vi "GDSLvIcon_BuildPictureRows.vi"(1 "RowTextPictures":cluster{"RowPict":bool[][]}[](array[cluster])=[{"RowPict"=[[FALSE, TRUE, TRUE, TRUE, FALSE, TRUE, TRUE, FALSE, FALSE, TRUE, FALSE], [TRUE, FALSE, FALSE, TRUE, FALSE, TRUE, FALSE, FALSE, FALSE, TRUE, FALSE], [TRUE, FALSE, TRUE, TRUE, FALSE, TRUE, TRUE, FALSE, FALSE, TRUE, FALSE], [TRUE, FALSE, FALSE, FALSE, FALSE, TRUE, FALSE, FALSE, FALSE, TRUE, FALSE], [FALSE, TRUE, TRUE, TRUE, FALSE, TRUE, TRUE, FALSE, TRUE, TRUE, TRUE]]}, {"RowPict"=[[TRUE, TRUE, FALSE, FALSE, TRUE, FALSE, TRUE, FALSE, FALSE, TRUE, FALSE, FALSE, TRUE, FALSE, TRUE], [TRUE, FALSE, TRUE, FALSE, TRUE, FALSE, TRUE, FALSE, FALSE, TRUE, FALSE, FALSE, TRUE, FALSE, TRUE], [TRUE, FALSE, TRUE, FALSE, TRUE, TRUE, TRUE, FALSE, FALSE, TRUE, FALSE, FALSE, TRUE, TRUE, TRUE], [TRUE, FALSE, TRUE, FALSE, TRUE, FALSE, TRUE, FALSE, FALSE, TRUE, FALSE, FALSE, TRUE, FALSE, TRUE], [TRUE, TRUE, FALSE, FALSE, FALSE, TRUE, FALSE, FALSE, TRUE, TRUE, TRUE, FALSE, FALSE, TRUE, FALSE]]}], 2 "Pixel width":i32=30, 3 "Alignment":T1, 4 "Offset":cluster{"X":i32, "Y":i32}, 5 "error in (no error)":errorcluster, 6 "Pixel height":i32=22) -> (15 "CharPicture":bool[][](array[boolean])=[[FALSE, FALSE, FALSE, FALSE, FALSE, FALSE, FALSE, FALSE, FALSE, FALSE, FALSE, FALSE, FALSE, FALSE, FALSE, FALSE, FALSE, FALSE, FALSE, FALSE, FALSE, FALSE, FALSE, FALSE, FALSE, FALSE, FALSE, FALSE, FALSE, FALSE], [FALSE, FALSE, FALSE, FALSE, FALSE, FALSE, FALSE, FALSE, FALSE, FALSE, FALSE, FALSE, FALSE, FALSE, FALSE, FALSE, FALSE, FALSE, FALSE, FALSE, FALSE, FALSE, FALSE, FALSE, FALSE, FALSE, FALSE, FALSE, FALSE, FALSE], [FALSE, FALSE, FALSE, FALSE, FALSE, FALSE, FALSE, FALSE, FALSE, FALSE, FALSE, FALSE, FALSE, FALSE, FALSE, FALSE, FALSE, FALSE, FALSE, FALSE, FALSE, FALSE, FALSE, FALSE, FALSE, FALSE, FALSE, FALSE, FALSE, FALSE], [FALSE, FALSE, FALSE, FALSE, FALSE, FALSE, FALSE, FALSE, FALSE, FALSE, FALSE, FALSE, FALSE, FALSE, FALSE, FALSE, FALSE, FALSE, FALSE, FALSE, FALSE, FALSE, FALSE, FALSE, FALSE, FALSE, FALSE, FALSE, FALSE, FALSE], [FALSE, FALSE, FALSE, FALSE, FALSE, FALSE, FALSE, FALSE, FALSE, FALSE, FALSE, FALSE, FALSE, FALSE, FALSE, FALSE, FALSE, FALSE, FALSE, FALSE, TRUE, TRUE, TRUE, FALSE, TRUE, TRUE, FALSE, TRUE, TRUE, TRUE], [FALSE, FALSE, FALSE, FALSE, FALSE, FALSE, FALSE, FALSE, FALSE, FALSE, FALSE, FALSE, FALSE, FALSE, FALSE, FALSE, FALSE, FALSE, FALSE, TRUE, FALSE, FALSE, FALSE, FALSE, TRUE, FALSE, FALSE, FALSE, TRUE, FALSE], [FALSE, FALSE, FALSE, FALSE, FALSE, FALSE, FALSE, FALSE, FALSE, FALSE, FALSE, FALSE, FALSE, FALSE, FALSE, FALSE, FALSE, FALSE, FALSE, TRUE, FALSE, TRUE, TRUE, FALSE, TRUE, TRUE, FALSE, FALSE, TRUE, FALSE], [FALSE, FALSE, FALSE, FALSE, FALSE, FALSE, FALSE, FALSE, FALSE, FALSE, FALSE, FALSE, FALSE, FALSE, FALSE, FALSE, FALSE, FALSE, FALSE, TRUE, FALSE, FALSE, TRUE, FALSE, TRUE, FALSE, FALSE, FALSE, TRUE, FALSE], [FALSE, FALSE, FALSE, FALSE, FALSE, FALSE, FALSE, FALSE, FALSE, FALSE, FALSE, FALSE, FALSE, FALSE, FALSE, FALSE, FALSE, FALSE, FALSE, FALSE, TRUE, TRUE, TRUE, FALSE, TRUE, TRUE, FALSE, FALSE, TRUE, FALSE], [FALSE, FALSE, FALSE, FALSE, FALSE, FALSE, FALSE, FALSE, FALSE, FALSE, FALSE, FALSE, FALSE, FALSE, FALSE, FALSE, FALSE, FALSE, FALSE, FALSE, FALSE, FALSE, FALSE, FALSE, FALSE, FALSE, FALSE, FALSE, FALSE, FALSE], [FALSE, FALSE, FALSE, FALSE, FALSE, FALSE, FALSE, FALSE, FALSE, FALSE, FALSE, FALSE, FALSE, FALSE, FALSE, FALSE, FALSE, FALSE, FALSE, FALSE, FALSE, FALSE, FALSE, FALSE, FALSE, FALSE, FALSE, FALSE, FALSE, FALSE], [FALSE, FALSE, FALSE, FALSE, FALSE, FALSE, FALSE, FALSE, FALSE, FALSE, FALSE, FALSE, FALSE, FALSE, FALSE, FALSE, FALSE, FALSE, FALSE, FALSE, FALSE, FALSE, FALSE, FALSE, FALSE, FALSE, FALSE, FALSE, FALSE, FALSE], [FALSE, FALSE, FALSE, FALSE, FALSE, FALSE, FALSE, FALSE, FALSE, FALSE, FALSE, FALSE, FALSE, FALSE, FALSE, FALSE, FALSE, FALSE, FALSE, FALSE, FALSE, FALSE, FALSE, FALSE, FALSE, FALSE, FALSE, FALSE, FALSE, FALSE], [FALSE, FALSE, FALSE, FALSE, FALSE, FALSE, FALSE, FALSE, FALSE, FALSE, FALSE, FALSE, FALSE, FALSE, FALSE, TRUE, TRUE, FALSE, FALSE, FALSE, TRUE, FALSE, FALSE, TRUE, TRUE, TRUE, FALSE, FALSE, TRUE, FALSE], [FALSE, FALSE, FALSE, FALSE, FALSE, FALSE, FALSE, FALSE, FALSE, FALSE, FALSE, FALSE, FALSE, FALSE, FALSE, TRUE, FALSE, TRUE, FALSE, TRUE, FALSE, TRUE, FALSE, FALSE, TRUE, FALSE, FALSE, TRUE, FALSE, TRUE], [FALSE, FALSE, FALSE, FALSE, FALSE, FALSE, FALSE, FALSE, FALSE, FALSE, FALSE, FALSE, FALSE, FALSE, FALSE, TRUE, FALSE, TRUE, FALSE, TRUE, TRUE, TRUE, FALSE, FALSE, TRUE, FALSE, FALSE, TRUE, TRUE, TRUE], [FALSE, FALSE, FALSE, FALSE, FALSE, FALSE, FALSE, FALSE, FALSE, FALSE, FALSE, FALSE, FALSE, FALSE, FALSE, TRUE, FALSE, TRUE, FALSE, TRUE, FALSE, TRUE, FALSE, FALSE, TRUE, FALSE, FALSE, TRUE, FALSE, TRUE], [FALSE, FALSE, FALSE, FALSE, FALSE, FALSE, FALSE, FALSE, FALSE, FALSE, FALSE, FALSE, FALSE, FALSE, FALSE, TRUE, TRUE, FALSE, FALSE, TRUE, FALSE, TRUE, FALSE, FALSE, TRUE, FALSE, FALSE, TRUE, FALSE, TRUE], [FALSE, FALSE, FALSE, FALSE, FALSE, FALSE, FALSE, FALSE, FALSE, FALSE, FALSE, FALSE, FALSE, FALSE, FALSE, FALSE, FALSE, FALSE, FALSE, FALSE, FALSE, FALSE, FALSE, FALSE, FALSE, FALSE, FALSE, FALSE, FALSE, FALSE], [FALSE, FALSE, FALSE, FALSE, FALSE, FALSE, FALSE, FALSE, FALSE, FALSE, FALSE, FALSE, FALSE, FALSE, FALSE, FALSE, FALSE, FALSE, FALSE, FALSE, FALSE, FALSE, FALSE, FALSE, FALSE, FALSE, FALSE, FALSE, FALSE, FALSE], [FALSE, FALSE, FALSE, FALSE, FALSE, FALSE, FALSE, FALSE, FALSE, FALSE, FALSE, FALSE, FALSE, FALSE, FALSE, FALSE, FALSE, FALSE, FALSE, FALSE, FALSE, FALSE, FALSE, FALSE, FALSE, FALSE, FALSE, FALSE, FALSE, FALSE], [FALSE, FALSE, FALSE, FALSE, FALSE, FALSE, FALSE, FALSE, FALSE, FALSE, FALSE, FALSE, FALSE, FALSE, FALSE, FALSE, FALSE, FALSE, FALSE, FALSE, FALSE, FALSE, FALSE, FALSE, FALSE, FALSE, FALSE, FALSE, FALSE, FALSE]], 17 "X-Limited":bool, 18 "Y-Limited":bool, 19 "error out":errorcluster)   [LabVIEW 2020]
doc: "Puts the separate rows together to one picture. Each row is center and filled with spaces in the beginning and end."
uses:
  <resource>/Framework/Providers/Open_GDS/ClassProviders/Common/LvIcon_class/GDSLvIcon_TextAlignment.ctl
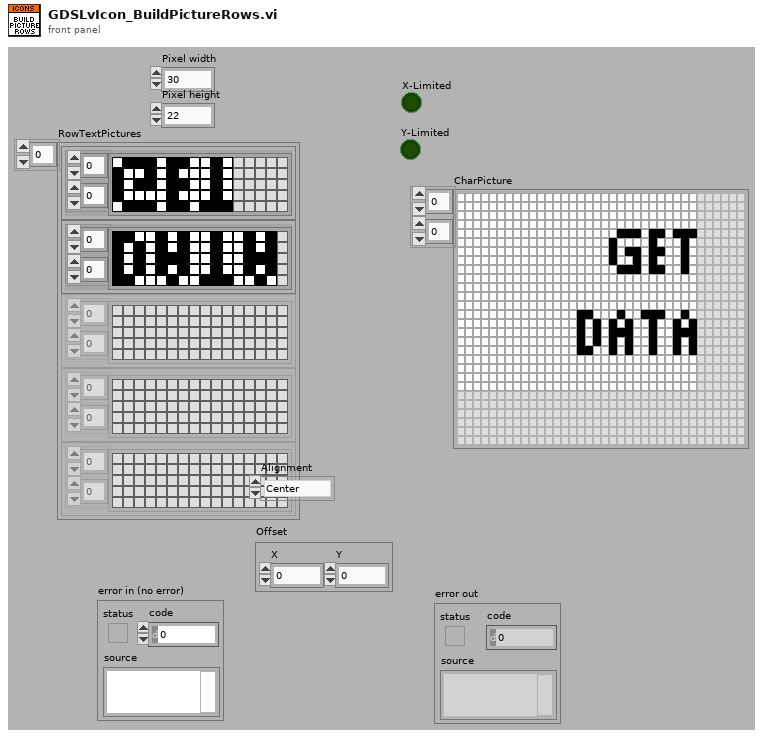
[diagram p1: front panel]
types:
  T1 = typedef "GDSLvIcon_TextAlignment.ctl" = enum16{"Center", "Left", "Right"}
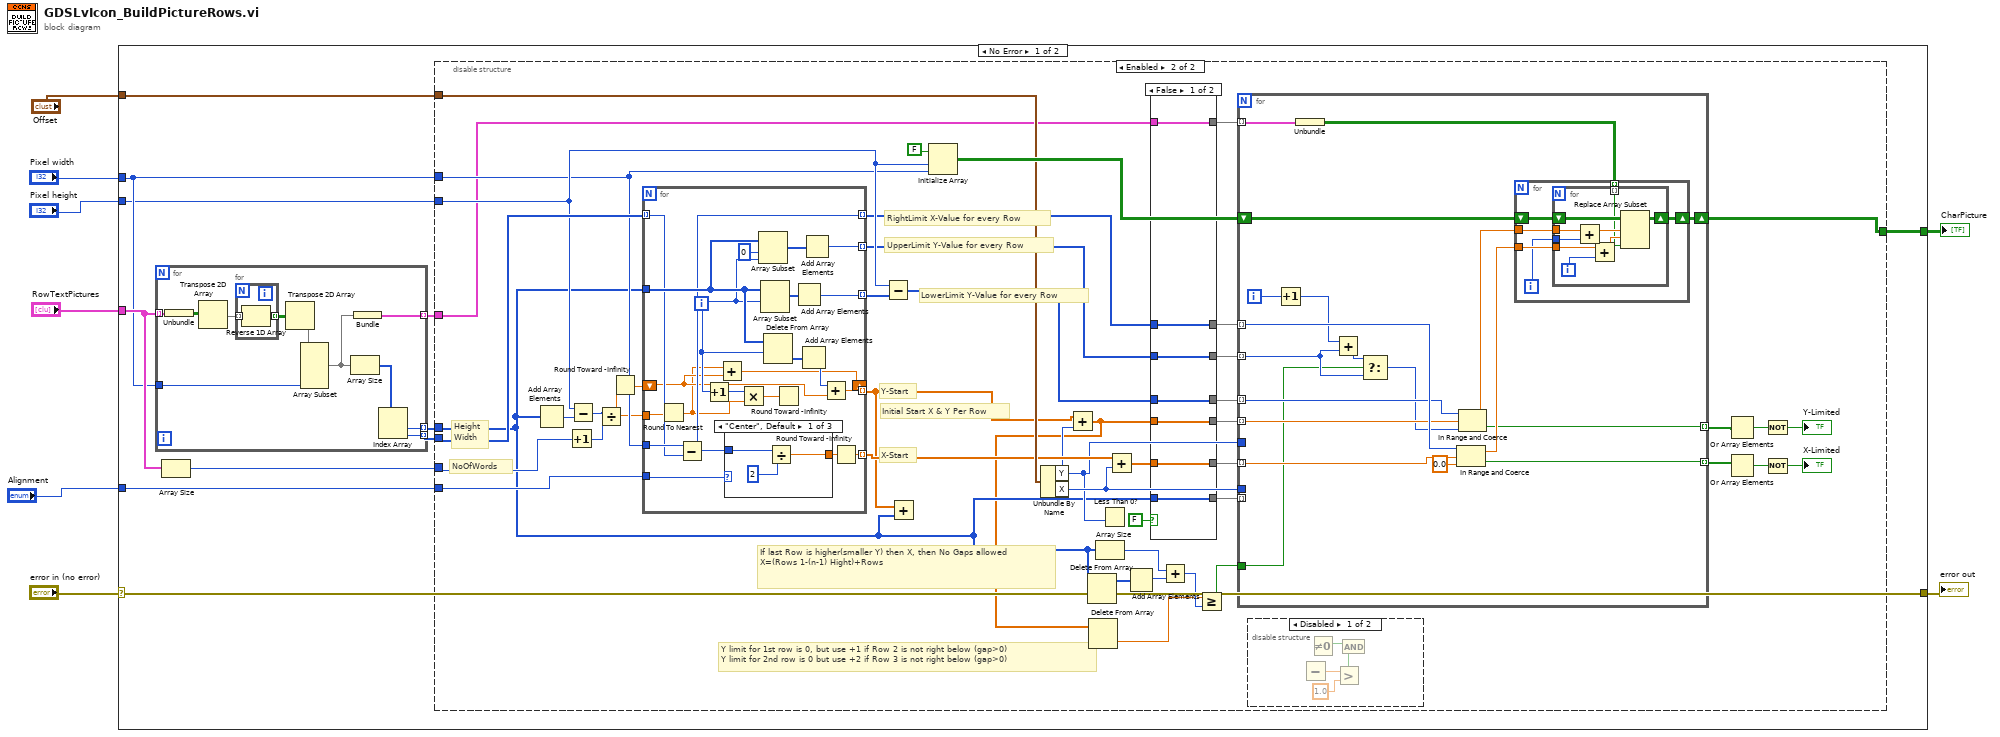
[diagram p0: block diagram]
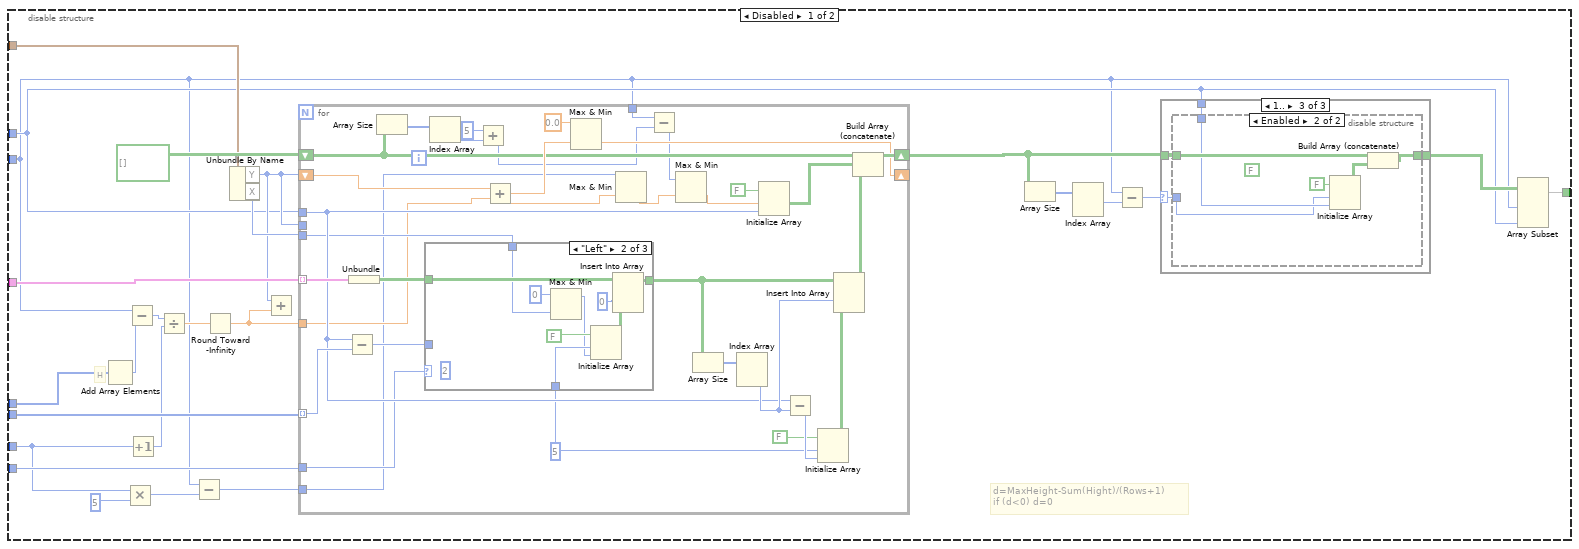
[diagram p2: hidden frame]
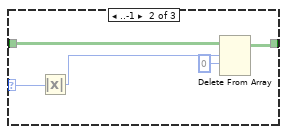
[diagram p4: hidden frame]
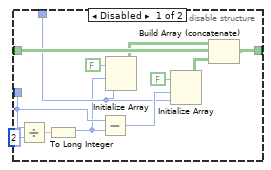
[diagram p5: hidden frame]
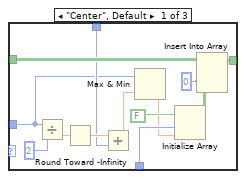
[diagram p6: hidden frame]
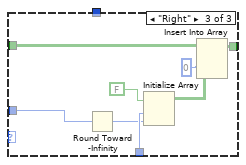
[diagram p7: hidden frame]
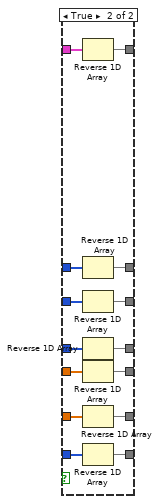
[diagram p9: hidden frame]
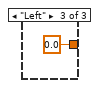
[diagram p11: hidden frame]
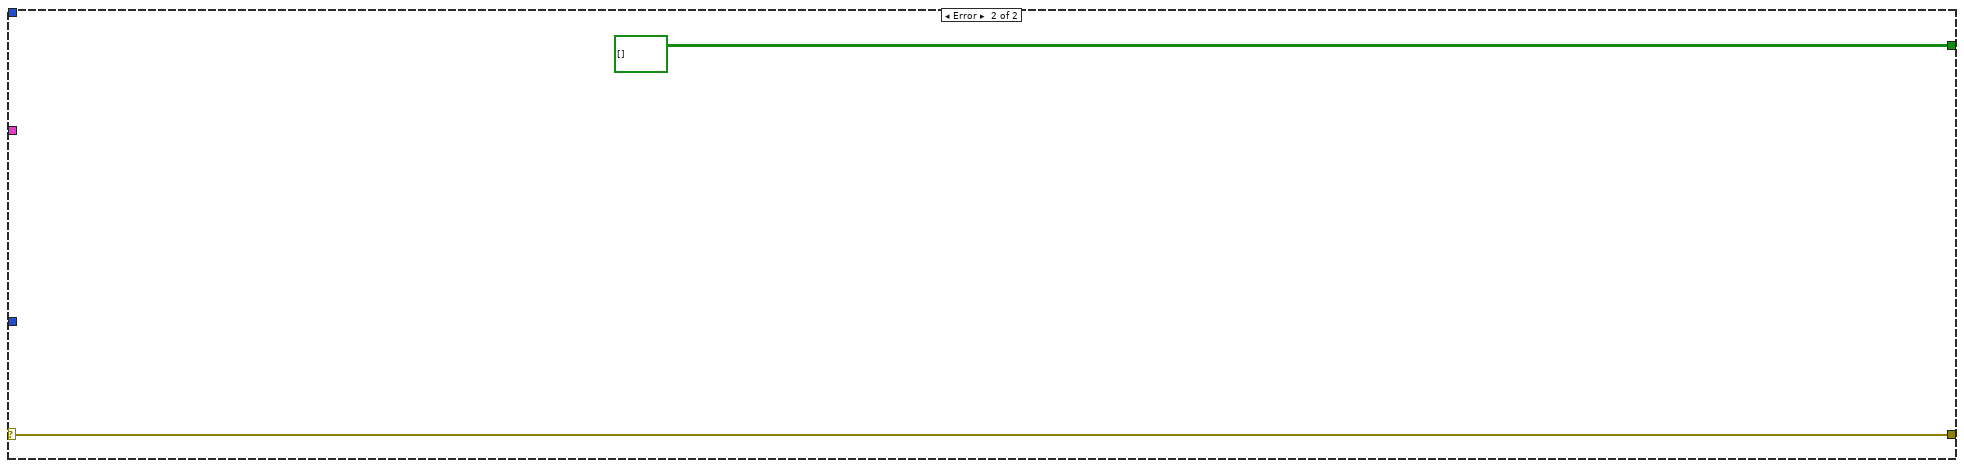
[diagram p12: hidden frame]
diagram:
  n1 = case shown="No Error" "error in (no error)" {
    selector: "error in (no error)" -> [w19 w282]
    tunnel: [w19 w282] -> w7
    tunnel: "Pixel width" -> [w11 _]
    tunnel: "RowTextPictures" -> [w15 _]
    tunnel: [w14 bool[][] [] ("CharPicture")] -> w5
    tunnel: "Pixel height" -> [w9 _]
    tunnel: "Alignment" -> [w13 _]
    tunnel: "Offset" -> [w12 _]
    frame No Error {
      n2 = for {
        tunnel: w15 -> [w275] mode=indexing
        tunnel: [w274] -> w17 mode=indexing
        tunnel: w11 -> [w273]
        tunnel: [w269] -> w18 mode=indexing
        tunnel: [w268] -> w16 mode=indexing
        n3 = Unbundle(w275) -> ("RowPict"=w276:bool[][])
        n4 = Transpose 2D Array(2D array=w276) -> (transposed array=w278:bool[][])
        n5 = for {
          tunnel: w278 -> [w280] mode=indexing
          tunnel: [w279] -> w277 mode=indexing
          n6 = Reverse 1D Array(array=w280) -> (reversed array=w279:bool[])
        }
        n7 = Transpose 2D Array(2D array=w277) -> (transposed array=w272:bool[][])
        n8 = Array Subset(array=w272, length (col)=w273) -> (w271:bool[][])  [unwired: 3 in]
        n9 = Array Size(array=w271) -> (size(s)=w270:i32[])
        n10 = Bundle(w271) -> (w274:cluster{bool[][]})  [unwired: 1 in]
        n11 = Index Array(array=w270) -> (element #1=w269:i32, element #2=w268:i32)  [unwired: 2 in]
      }
      n12 = Array Size(array=w15) -> (size(s)=w10:i32)
      n13 = disable-structure shown="Enabled" {
        disable-tunnel: w18 -> [w44 w140]
        disable-tunnel: w17 -> [w43 w156]
        disable-tunnel: w16 -> [w41 w178]
        disable-tunnel: [w37 w170] -> w14
        disable-tunnel: w13 -> [w36 w177]
        disable-tunnel: w12 -> [w34 w171]
        disable-tunnel: w11 -> [w25 w173]
        disable-tunnel: w10 -> [w23 w169]
        disable-tunnel: w9 -> [w20 w174]
        frame Disabled {
          # "d=MaxHeight-Sum(Hight)/(Rows+1)\nif (d<0) d=0"
          # "H"
          n14 = Add Array Elements(numeric array=w44) -> (sum=w40:i32)
          n15 = Multiply(x=w23, y=5 ("Disabled Index (col)")) -> (x*y=w22:i32)
          n16 = Subtract(x=w20, y=w40) -> (x-y=w39:i32)
          n17 = Increment(x=w23) -> (x+1=w38:i32)
          n18 = Divide(x=w39, y=w38) -> (x/y=w33:dbl)
          n19 = Subtract(x=w20, y=w22) -> (x-y=w21:i32)
          n20 = Round Toward -Infinity(1:w33) -> (0:w32:dbl)
          n21 = Unbundle By Name(w34) -> ("Y"=w31:i32, "X"=w35:i32)
          n22 = Add(x=w31, y=w32) -> ()  [unwired: 1 out]
          n23 = for {
            tunnel: w43 -> [w105] mode=indexing
            shift-right: [w101] -> w27
            shift-left: bool[][] [] ("CharPicture") -> [w81]
            tunnel: w41 -> [w104] mode=indexing
            tunnel: w25 -> [w92]
            tunnel: w32 -> [w87]
            tunnel: w36 -> [w91]
            tunnel: w35 -> [w90]
            tunnel: w31 -> [_]
            shift-right: [w85] -> _
            shift-left: w31 -> [w88]
            tunnel: w21 -> [w82]
            tunnel: w20 -> [w75]
            w83 = 5 ("Disabled Index (col)")
            n24 = Subtract(x=w92, y=w104) -> (x-y=w103:i32)
            n25 = Unbundle(w105) -> (w102:bool[][])
            n26 = Array Size(array=w81) -> (size(s)=w80:i32[])
            n27 = case shown="\"Left\"" w91 {
              tunnel: w103 -> [w106 _ w128]
              tunnel: w102 -> [w117 w127 w135]
              tunnel: [w113 w124 w132] -> w99
              tunnel: w83 -> [w112 w123 w131]
              tunnel: w90 -> [w109 w119 _]
              frame "Center", Default {
                n28 = Divide(x=w106, y=2) -> (x/y=w114:dbl)
                n29 = Round Toward -Infinity(1:w114) -> (0:w110:dbl)
                n30 = Add(x=w110, y=w109) -> (x+y=w107:dbl)
                n31 = Max & Min(x=w106, y=w107) -> (min(x,y)=w108:dbl)  [unwired: 1 out]
                n32 = Initialize Array(FALSE, w112, w108) -> (w115:bool[][])
                n33 = Insert Into Array(array=w117, index (col)=0 ("Disabled Index (col)"), new element=w115) -> (w113:bool[][])  [unwired: 1 in]
              }
              frame "Left" {
                (unwired) 2 ("y")
                n34 = Max & Min(x=0, y=w119) -> (max(x,y)=w120:i32)  [unwired: 1 out]
                n35 = Initialize Array(FALSE, w123, w120) -> (w125:bool[][])
                n36 = Insert Into Array(array=w127, index (col)=0 ("Disabled Index (col)"), new element=w125) -> (w124:bool[][])  [unwired: 1 in]
              }
              frame "Right" {
                n37 = Round Toward -Infinity(1:w128) -> (0:w130:i32)
                n38 = Initialize Array(FALSE, w131, w130) -> (w133:bool[][])
                n39 = Insert Into Array(array=w135, index (col)=0 ("Disabled Index (col)"), new element=w133) -> (w132:bool[][])  [unwired: 1 in]
              }
            }
            n40 = Index Array(array=w80) -> (element=w79:i32)  [unwired: 1 in]
            n41 = Add(x=5, y=w79) -> (x+y=w74:i32)
            n42 = Add(x=w88, y=w87) -> (x+y=w84:dbl)
            n43 = Max & Min(x=0.0, y=w84) -> (min(x,y)=w85:dbl)  [unwired: 1 out]
            n44 = Max & Min(x=w82, y=w84) -> (min(x,y)=w77:dbl)  [unwired: 1 out]
            n45 = Subtract(x=w75, y=w74) -> (x-y=w73:i32)
            n46 = Max & Min(x=w73, y=w77) -> (min(x,y)=w76:dbl)  [unwired: 1 out]
            n47 = Array Size(array=w99) -> (size(s)=w98:i32[])
            n48 = Index Array(array=w98) -> (element #2=w95:i32)  [unwired: 2 in, 1 out]
            n49 = Initialize Array(FALSE, w76, w92) -> (w89:bool[][])
            n50 = Subtract(x=w92, y=w95) -> (x-y=w96:i32)
            n51 = Initialize Array(FALSE, w83, w96) -> (w97:bool[][])
            n52 = Insert Into Array(array=w99, index (col)=w95, new element=w97) -> (w100:bool[][])  [unwired: 1 in]
            n53 = Build Array (concatenate)(w81, w89, w100) -> (w101:bool[][])
          }
          n54 = Array Size(array=w27) -> (size(s)=w30:i32[])
          n55 = Index Array(array=w30) -> (element #1=w29:i32)  [unwired: 2 in, 1 out]
          n56 = Subtract(x=w20, y=w29) -> (x-y=w28:i32)
          n57 = case shown="1.." w28 {
            selector: w28 -> [_ w50 w52]
            tunnel: w27 -> [w45 w49 w53]
            tunnel: [w45 w48 w54] -> w26
            tunnel: w25 -> [_ _ w51]
            frame Default {
            }
            frame ..-1 {
              n58 = Absolute Value(x=w50) -> (abs(x)=w46:i32)
              n59 = Delete From Array(array=w49, length=w46, index (row)=0) -> (array with subset deleted=w48:bool[][])  [unwired: 1 in, 1 out]
            }
            frame 1.. {
              n60 = disable-structure shown="Enabled" {
                disable-tunnel: [w66 w72] -> w54
                disable-tunnel: w53 -> [w63 w69]
                disable-tunnel: w52 -> [w60 w67]
                disable-tunnel: w51 -> [w57 w68]
                frame Disabled {
                  n61 = Divide(x=w60, y=2) -> (x/y=w61:dbl)
                  n62 = To Long Integer(number=w61) -> (32bit integer=w56:i32)
                  n63 = Subtract(x=w60, y=w56) -> (x-y=w59:i32)
                  n64 = Initialize Array(FALSE, w56, w57) -> (w55:bool[][])
                  n65 = Initialize Array(FALSE, w59, w57) -> (w64:bool[][])
                  n66 = Build Array (concatenate)(w55, w63, w64) -> (w66:bool[][])
                }
                frame Enabled {
                  (unwired) FALSE
                  n67 = Initialize Array(FALSE, w67, w68) -> (w70:bool[][])
                  n68 = Build Array (concatenate)(w69, w70) -> (w72:bool[][])
                }
              }
            }
          }
          n69 = Array Subset(array=w26, length (row)=w20, length (col)=w25) -> (w37:bool[][])  [unwired: 2 in]
        }
        frame Enabled {
          # "If last Row is higher(smaller Y) then X, then No Gaps allowed\nX=(Rows 1-(n-1) Hight)+Rows"
          # "Y limit for 1st row is 0, but use +1 if Row 2 is not right below (gap>0)\nY limit for 2nd row is 0 but use +2 if Row 3 is not right below (gap>0)"
          # "RightLimit X-Value for every Row"
          # "UpperLimit Y-Value for every Row"
          # "LowerLimit Y-Value for every Row"
          # "X-Start"
          # "Y-Start"
          # "Initial Start X & Y Per Row"
          # "NoOfWords"
          # "Height\nWidth"
          n70 = Add Array Elements(numeric array=w140) -> (sum=w181:i32)
          n71 = Increment(x=w169) -> (x+1=w179:i32)
          n72 = Subtract(x=w174, y=w181) -> (x-y=w180:i32)
          n73 = Divide(x=w180, y=w179) -> (x/y=w146:dbl)
          n74 = Round Toward -Infinity(1:w146) -> (0:w147:dbl)
          n75 = for {
            tunnel: w178 -> [w246] mode=indexing
            tunnel: w140 -> [w251]
            tunnel: [w256] -> w176 mode=indexing
            tunnel: [w259] -> w158 mode=indexing
            tunnel: [w245] -> w157 mode=indexing
            tunnel: w177 -> [w252]
            tunnel: w146 -> [w243]
            tunnel: [w255] -> w139 mode=indexing
            tunnel: w173 -> [w254]
            tunnel: [w247] -> w162 mode=indexing
            shift-right: [w242] -> _
            shift-left: w147 -> [w244]
            i -> [w250]
            n76 = Round To Nearest(number=w243) -> (nearest integer value=w241:dbl)
            n77 = Subtract(x=w254, y=w246) -> (x-y=w245:i32)
            n78 = Increment(x=w250) -> (x+1=w258:i32)
            n79 = Add(x=w241, y=w244) -> (x+y=w242:dbl)
            n80 = case shown="\"Center\", Default" w252 {
              tunnel: w245 -> [w265 w266 _]
              tunnel: [w263 w266 0.0] -> w253
              frame "Center", Default {
                n81 = Divide(x=w265, y=2) -> (x/y=w263:dbl)
              }
              frame "Right" {
              }
              frame "Left" {
              }
            }
            n82 = Multiply(x=w258, y=w241) -> (x*y=w257:dbl)
            n83 = Array Subset(array=w251, index=0, length=w250) -> (w260:i32[])
            n84 = Array Subset(array=w251, index=w250) -> (w262:i32[])  [unwired: 1 in]
            n85 = Delete From Array(array=w251, length=w250) -> (deleted portion=w249:i32[])  [unwired: 1 in, 1 out]
            n86 = Round Toward -Infinity(1:w257) -> ()  [unwired: 1 out]
            n87 = Add Array Elements(numeric array=w262) -> (sum=w256:i32)
            n88 = Add Array Elements(numeric array=w249) -> (sum=w248:i32)
            n89 = Add Array Elements(numeric array=w260) -> (sum=w259:i32)
            n90 = Add(x=w248, y=w244) -> (x+y=w255:dbl)
            n91 = Round Toward -Infinity(1:w253) -> (0:w247:dbl)
          }
          n92 = Subtract(x=w174, y=w176) -> (x-y=w159:i32[])
          n93 = Add(x=w139, y=w140) -> ()  [unwired: 1 out]
          n94 = Initialize Array(FALSE, w174, w173) -> (w172:bool[][])
          n95 = Unbundle By Name(w171) -> ("Y"=w160:i32, "X"=w161:i32)
          n96 = Add(x=w139, y=w160) -> (x+y=w138:dbl[])
          n97 = Delete From Array(array=w140) -> (array with subset deleted=w144:i32[])  [unwired: 2 in, 1 out]
          n98 = Delete From Array(array=w138) -> (deleted portion=w137:dbl)  [unwired: 2 in, 1 out]
          n99 = Array Size(array=w140) -> (size(s)=w142:i32)
          n100 = Less Than 0?(x=w160) -> ()  [unwired: 1 out]
          n101 = Add(x=w162, y=w161) -> (x+y=w151:dbl[])
          n102 = Add Array Elements(numeric array=w144) -> (sum=w143:i32)
          n103 = case shown="False" FALSE {
            tunnel: w140 -> [w187 w199]
            tunnel: w159 -> [w190 w202]
            tunnel: w158 -> [w191 w203]
            tunnel: w157 -> [w192 w204]
            tunnel: w156 -> [w186 w206]
            tunnel: [w192 w193] -> w155
            tunnel: [w191 w194] -> w154
            tunnel: [w190 w195] -> w153
            tunnel: w138 -> [w189 w201]
            tunnel: [w189 w196] -> w152
            tunnel: w151 -> [w188 w200]
            tunnel: [w188 w197] -> w150
            tunnel: [w187 w198] -> w149
            tunnel: [w186 w205] -> w148
            frame False {
            }
            frame True {
              n104 = Reverse 1D Array(array=w206) -> (reversed array=w205:cluster{bool[][]}[])
              n105 = Reverse 1D Array(array=w204) -> (reversed array=w193:i32[])
              n106 = Reverse 1D Array(array=w203) -> (reversed array=w194:i32[])
              n107 = Reverse 1D Array(array=w202) -> (reversed array=w195:i32[])
              n108 = Reverse 1D Array(array=w201) -> (reversed array=w196:dbl[])
              n109 = Reverse 1D Array(array=w200) -> (reversed array=w197:dbl[])
              n110 = Reverse 1D Array(array=w199) -> (reversed array=w198:i32[])
            }
          }
          n111 = Add(x=w142, y=w143) -> (x+y=w141:i32)
          n112 = Greater Or Equal?(x=w137, y=w141) -> (x >= y?=w136:bool)
          n113 = for {
            shift-right: [w225] -> w170
            shift-left: w172 -> [w224]
            tunnel: w153 -> [w215] mode=indexing
            tunnel: w154 -> [w211] mode=indexing
            tunnel: w155 -> [w223] mode=indexing
            tunnel: w160 -> [_]
            tunnel: w161 -> [_]
            tunnel: w148 -> [w220] mode=indexing
            tunnel: [w218] -> w168 mode=indexing
            tunnel: [w217] -> w163 mode=indexing
            tunnel: w152 -> [w212] mode=indexing
            tunnel: w150 -> [w216] mode=indexing
            tunnel: w149 -> [_] mode=indexing
            tunnel: w136 -> [w207]
            i -> [w210]
            n114 = Increment(x=w210) -> (x+1=w209:i32)
            n115 = Unbundle(w220) -> (w219:bool[][])
            n116 = Add(x=w209, y=w211) -> (x+y=w214:i32)
            n117 = Select(t=w214, s=w207, f=w211) -> (s? t:f=w208:i32)
            n118 = In Range and Coerce(upper limit=w223, x=w216, lower limit=0.0) -> (coerced(x)=w221:dbl, In Range?=w217:bool)
            n119 = In Range and Coerce(upper limit=w215, x=w212, lower limit=w208) -> (coerced(x)=w213:dbl, In Range?=w218:bool)
            n120 = for {
              tunnel: w213 -> [w230]
              tunnel: w221 -> [w229]
              shift-right: [w231] -> w225
              shift-left: w224 -> [w228]
              tunnel: w219 -> [w227] mode=indexing
              i -> [w226]
              n121 = for {
                tunnel: w230 -> [w238]
                tunnel: w229 -> [w236]
                shift-right: [w240] -> w231
                shift-left: w228 -> [w239]
                tunnel: w227 -> [w234] mode=indexing
                tunnel: w226 -> [w233]
                i -> [w232]
                n122 = Add(x=w238, y=w233) -> (x+y=w237:dbl)
                n123 = Add(x=w236, y=w232) -> (x+y=w235:dbl)
                n124 = Replace Array Subset(array=w239, new element=w234, index (row)=w237, index (col)=w235) -> (w240:bool[][])
              }
            }
          }
          n125 = disable-structure shown="Disabled" {
            frame Disabled {
              n126 = Subtract() -> (x-y=w182:dbl)  [unwired: 2 in]
              n127 = Not Equal To 0?() -> (x != 0?=w184:bool)  [unwired: 1 in]
              n128 = Greater?(x=w182, y=1.0) -> (0:w185:bool)
              n129 = And(x=w184, y=w185) -> ()  [unwired: 1 out]
            }
            frame Enabled {
            }
          }
          n130 = Or Array Elements(Boolean array=w168) -> (logical OR=w167:bool)
          n131 = Or Array Elements(Boolean array=w163) -> (logical OR=w164:bool)
          n132 = Not(x=w167) -> (.not. x?=→"Y-Limited":bool)
          n133 = Not(x=w164) -> (.not. x?=→"X-Limited":bool)
        }
      }
    }
    frame Error {
    }
  }
  "error out" <- w7
  "CharPicture" <- w5
